vi "ZeroPadCDB.vi"(5 "Input Array":cdb[](array[numeric]) format="%.2f", 6 "FFT size":u16(ring) items=["next 2^n", "8", "16", "32", "64", "128", "256", "512"]) -> (1 "Length of padded array":i32, 2 "Ouput Array":cdb[](array[numeric]) format="%.2f")   [LabVIEW 2022 SP3]
uses:
  <vilib>/Analysis/2dsp.llb/Zero Padder (CDB).vi
  <vilib>/Analysis/NI_AALPro.lvlib
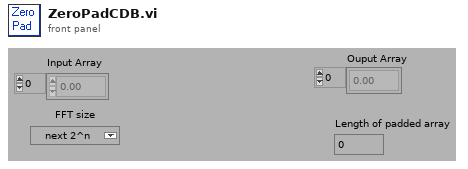
[diagram p1: front panel]
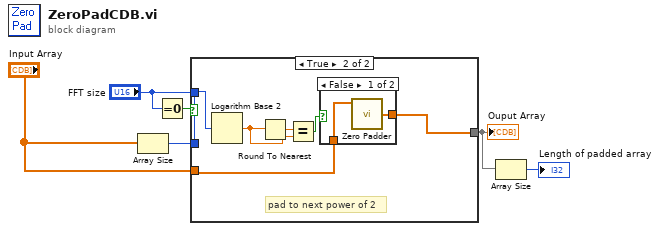
[diagram p0: block diagram]
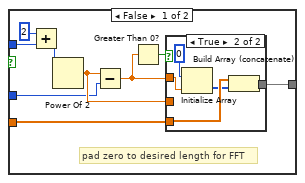
[diagram p2: hidden frame]
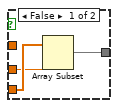
[diagram p3: hidden frame]
diagram:
  n1 = Array Size(array="Input Array") -> (size(s)=w4:i32)
  n2 = Equal To 0?(x="FFT size") -> (x = 0?=w6:bool)
  n3 = case shown="True" w6 {
    tunnel: "FFT size" -> [w13 _]
    tunnel: "Input Array" -> [w11 w26]
    tunnel: w4 -> [w8 w24]
    tunnel: [w7 w25] -> w2
    frame False {
      # "pad zero to desired length for FFT"
      n4 = Add(x=u16 2, y=w13) -> (x+y=w15:u16)
      n5 = Power Of 2(x=w15) -> (2^x=w9:dbl)
      n6 = Subtract(x=w9, y=w8) -> (x-y=w12:dbl)
      n7 = Greater Than 0?(x=w12) -> (x > 0?=w10:bool)
      n8 = case shown="True" w10 {
        tunnel: w12 -> [_ w20]
        tunnel: w11 -> [w18 w23]
        tunnel: w9 -> [w17 _]
        tunnel: [w16 w22] -> w7
        frame False {
          n9 = Array Subset(array=w18, length=w17) -> (w16:cdb[])  [unwired: 1 in]
        }
        frame True {
          n10 = Initialize Array(0 ("Dimension Size"), w20) -> (w19:i32[])
          n11 = Build Array (concatenate)(w23, w19) -> (w22:cdb[])
        }
      }
    }
    frame True {
      # "pad to next power of 2"
      n12 = Logarithm Base 2(1:w24) -> (0:w28:dbl)
      n13 = Round To Nearest(number=w28) -> (nearest integer value=w29:dbl)
      n14 = Equal?(x=w29, y=w28) -> (x = y?=w27:bool)
      n15 = case shown="False" w27 {
        tunnel: w26 -> [w31 w32]
        tunnel: [w30 w32] -> w25
        frame False {
          n16 = call-poly <vilib>:"Zero Padder.vi"("Input Array"=w31) -> ("Zero Padded Array"=w30:cdb[])  [unwired: 1 in, 9 out]
        }
        frame True {
        }
      }
    }
  }
  "Ouput Array" <- w2
  n17 = Array Size(array=w2) -> (size(s)=→"Length of padded array":i32)
